vi "writegraph_OLD.vi"(4 "Numeric":i16, 5 "Array":string[][](array[string])) -> ()   [LabVIEW 2011]
uses:
  Dependencies/global.vi
panel:
  out "Humidity (Mote 1001)":dbl(graph)
  out "Temperature (Mote 1001)":dbl(graph)
  out "CO2 (Mote 1001)":dbl(graph)
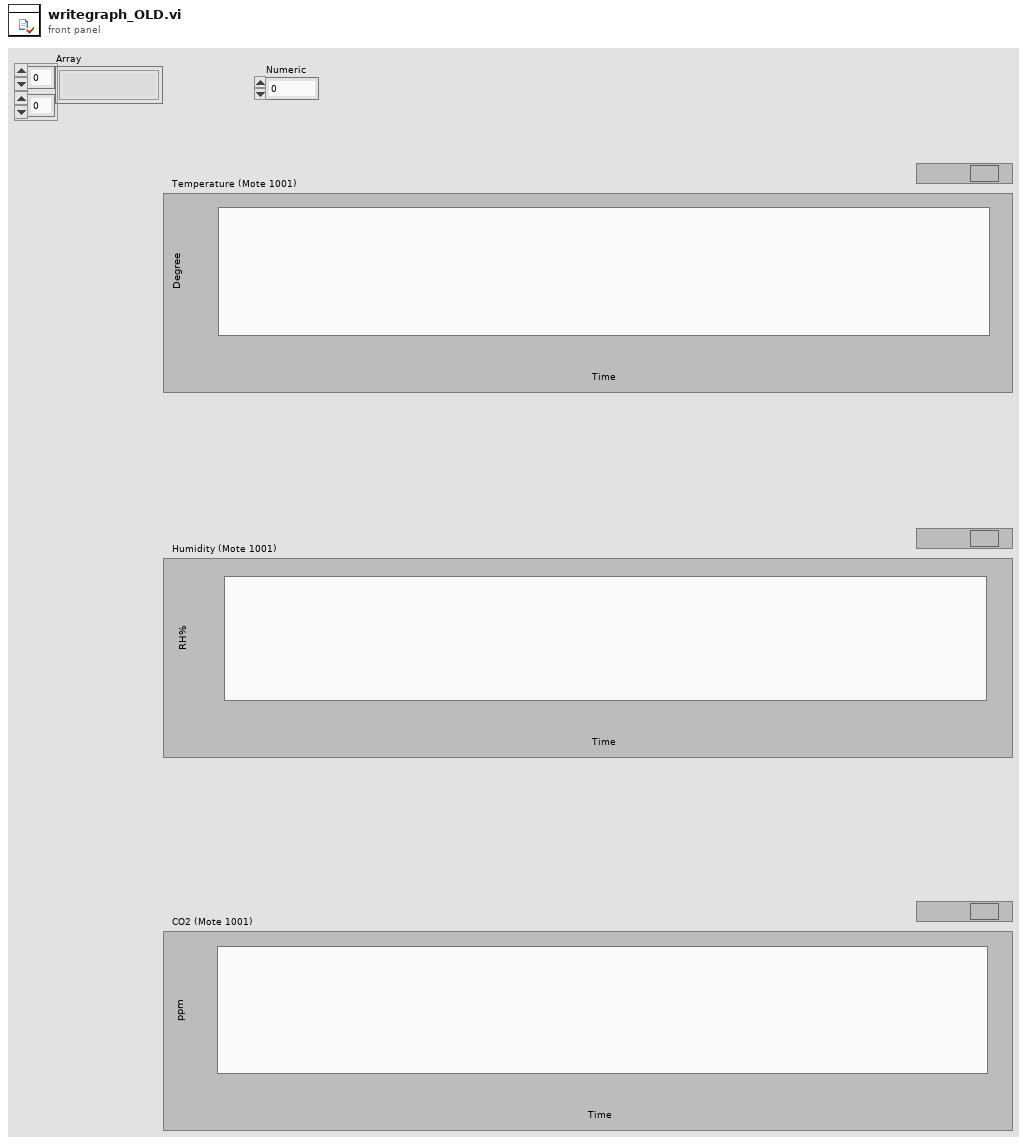
[diagram p1: front panel]
types:
  T1 = typedef "imagedata.ctl" = cluster{"image type":i32, "image depth":i32, "image":u8[], "mask":u8[], "colors":u32[], "Rectangle":cluster{"left":i16, "top":i16, "right":i16, "bottom":i16}}
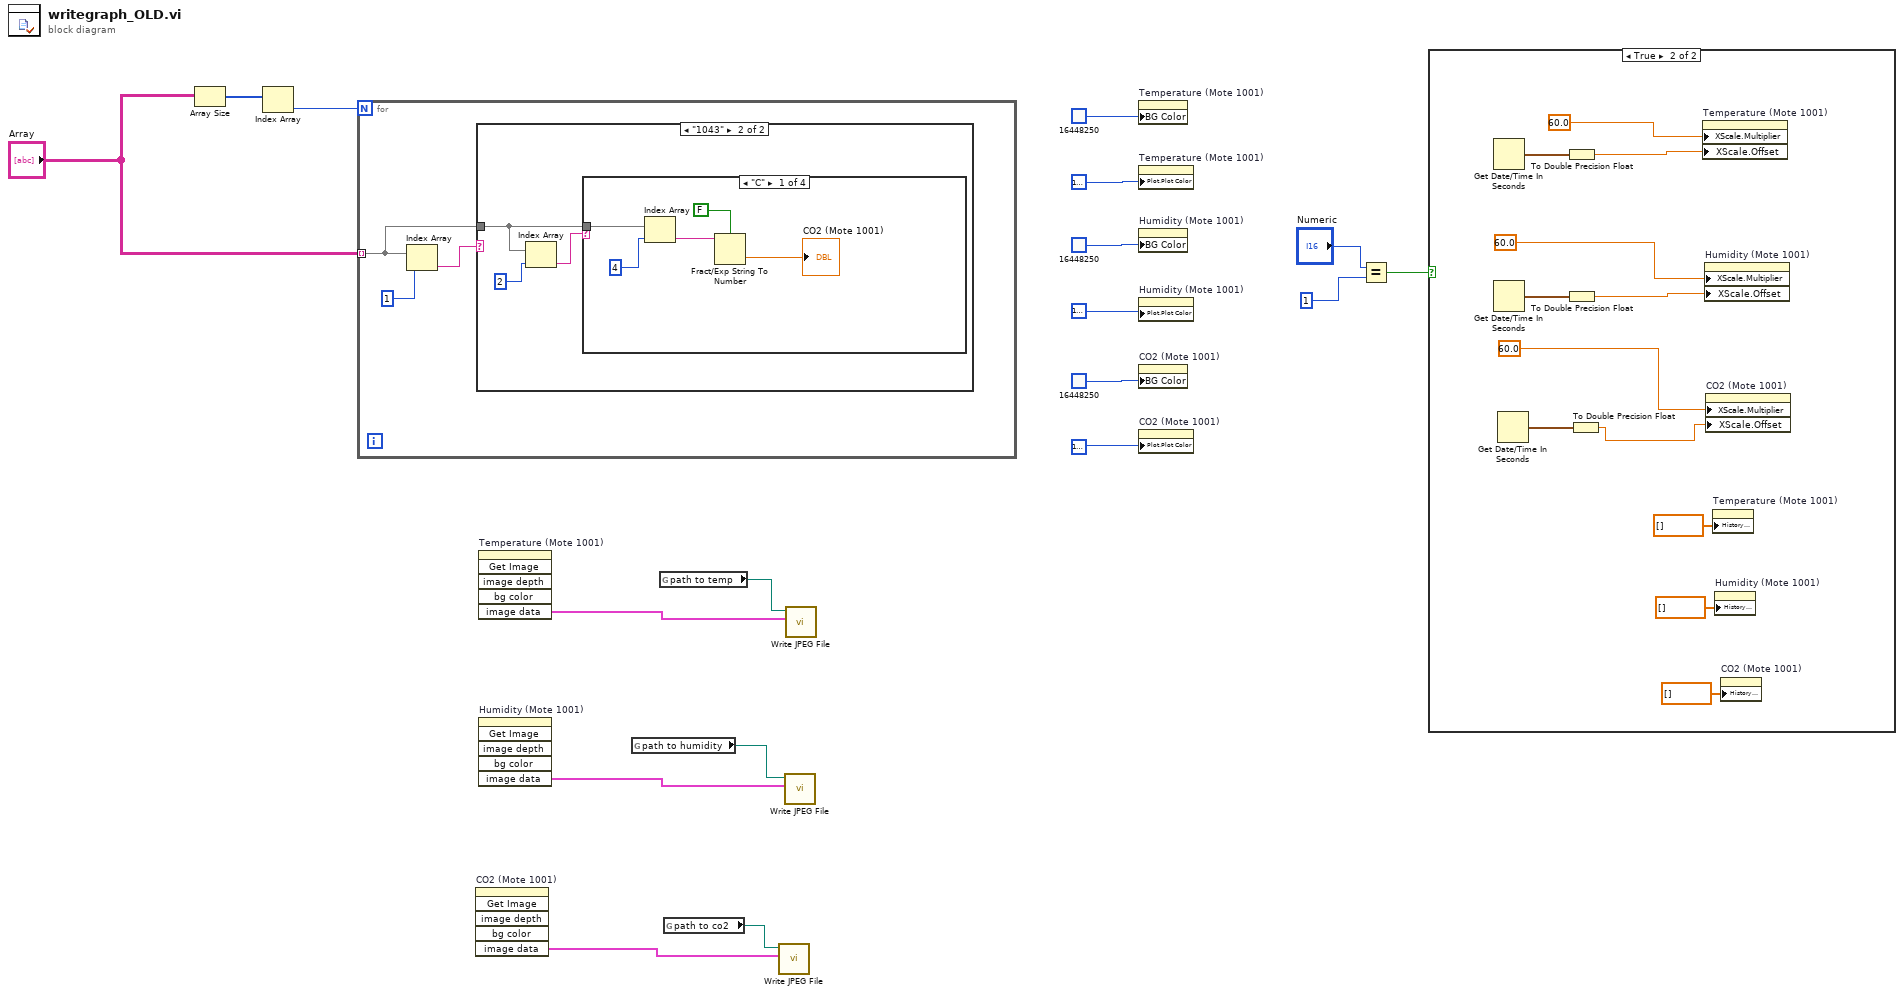
[diagram p0: block diagram]
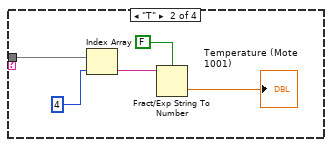
[diagram p4: hidden frame]
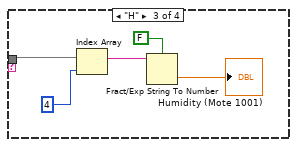
[diagram p5: hidden frame]
diagram:
  n1 = Array Size(array="Array") -> (size(s)=w18:i32[])
  n2 = Index Array(array=w18) -> (element=w17:i32)  [unwired: 1 in]
  n3 = for {
    N: w17 -> [_]
    tunnel: "Array" -> [w19] mode=indexing
    n4 = Index Array(array=w19, index=1) -> (element=w20:string)
    n5 = case shown="\"1043\"" w20 {
      tunnel: w19 -> [_ w24]
      frame "0", Default {
      }
      frame "1043" {
        n6 = Index Array(array=w24, index=2) -> (element=w22:string)
        n7 = case shown="\"C\"" w22 {
          tunnel: w24 -> [w27 w34 w37 _]
          frame "C" {
            n8 = Index Array(array=w27, index=4 ("index (row)")) -> (element=w28:string)
            n9 = Fract/Exp String To Number(use system decimal point (T)=FALSE, string=w28) -> (number=→"CO2 (Mote 1001)":dbl)  [unwired: 2 in, 1 out]
          }
          frame "T" {
            n10 = Index Array(array=w34, index=4 ("index (row)")) -> (element=w32:string)
            n11 = Fract/Exp String To Number(use system decimal point (T)=FALSE, string=w32) -> (number=→"Temperature (Mote 1001)":dbl)  [unwired: 2 in, 1 out]
          }
          frame "H" {
            n12 = Index Array(array=w37, index=4 ("index (row)")) -> (element=w38:string)
            n13 = Fract/Exp String To Number(use system decimal point (T)=FALSE, string=w38) -> (number=→"Humidity (Mote 1001)":dbl)  [unwired: 2 in, 1 out]
          }
          frame Default {
          }
        }
      }
    }
  }
  n14 = invoke on="CO2 (Mote 1001)" class="WFChart (strict)" method="Get Image"() -> ("image data"=w7:T1)  [unwired: 6 in, 5 out]
  n15 = invoke on="Temperature (Mote 1001)" class="WFChart (strict)" method="Get Image"() -> ("image data"=w9:T1)  [unwired: 6 in, 5 out]
  n16 = invoke on="Humidity (Mote 1001)" class="WFChart (strict)" method="Get Image"() -> ("image data"=w8:T1)  [unwired: 6 in, 5 out]
  n17 = global read "global.vi" "path to humidity"() -> (w2:path)
  n18 = global read "global.vi" "path to temp"() -> (w1:path)
  n19 = global read "global.vi" "path to co2"() -> (w3:path)
  n20 = call <vilib>:"Write JPEG File.vi"("image data"=w7, "path to JPEG file"=w3) -> ()  [unwired: 8 in, 2 out]
  n21 = call <vilib>:"Write JPEG File.vi"("image data"=w8, "path to JPEG file"=w2) -> ()  [unwired: 8 in, 2 out]
  n22 = call <vilib>:"Write JPEG File.vi"("image data"=w9, "path to JPEG file"=w1) -> ()  [unwired: 8 in, 2 out]
  n23 = property on="Temperature (Mote 1001)" class="WFChart (strict)"("BG Color"=u32 16448250) -> ()  [unwired: 2 in, 2 out]
  n24 = property on="Temperature (Mote 1001)" class="WFChart (strict)"("Plot.Plot Color"=u32 16777222) -> ()  [unwired: 2 in, 2 out]
  n25 = property on="Humidity (Mote 1001)" class="WFChart (strict)"("BG Color"=u32 16448250) -> ()  [unwired: 2 in, 2 out]
  n26 = property on="Humidity (Mote 1001)" class="WFChart (strict)"("Plot.Plot Color"=u32 16777222) -> ()  [unwired: 2 in, 2 out]
  n27 = property on="CO2 (Mote 1001)" class="WFChart (strict)"("BG Color"=u32 16448250) -> ()  [unwired: 2 in, 2 out]
  n28 = property on="CO2 (Mote 1001)" class="WFChart (strict)"("Plot.Plot Color"=u32 16777222) -> ()  [unwired: 2 in, 2 out]
  n29 = Equal?(x="Numeric", y=i16 1) -> (x = y?=w6:bool)
  n30 = case shown="True" w6 {
    frame False {
    }
    frame True {
      n31 = Get Date/Time In Seconds() -> (seconds since 1Jan1904=w51:timestamp)
      n32 = Get Date/Time In Seconds() -> (seconds since 1Jan1904=w50:timestamp)
      n33 = Get Date/Time In Seconds() -> (seconds since 1Jan1904=w48:timestamp)
      n34 = To Double Precision Float(number=w51) -> (double precision float=w45:dbl)
      n35 = To Double Precision Float(number=w50) -> (double precision float=w44:dbl)
      n36 = To Double Precision Float(number=w48) -> (double precision float=w43:dbl)
      n37 = property on="Temperature (Mote 1001)" class="WFChart (strict)"("XScale.Multiplier"=60.0 ("X Scale.Offset and Multiplier:Multiplier"), "XScale.Offset"=w45) -> ()  [unwired: 2 in, 2 out]
      n38 = property on="Humidity (Mote 1001)" class="WFChart (strict)"("XScale.Multiplier"=60.0 ("X Scale.Offset and Multiplier:Multiplier"), "XScale.Offset"=w44) -> ()  [unwired: 2 in, 2 out]
      n39 = property on="CO2 (Mote 1001)" class="WFChart (strict)"("XScale.Multiplier"=60.0 ("X Scale.Offset and Multiplier:Multiplier"), "XScale.Offset"=w43) -> ()  [unwired: 2 in, 2 out]
      n40 = property on="Temperature (Mote 1001)" class="WFChart (strict)"("History Data"=dbl[] []) -> ()  [unwired: 2 in, 2 out]
      n41 = property on="Humidity (Mote 1001)" class="WFChart (strict)"("History Data"=dbl[] []) -> ()  [unwired: 2 in, 2 out]
      n42 = property on="CO2 (Mote 1001)" class="WFChart (strict)"("History Data"=dbl[] []) -> ()  [unwired: 2 in, 2 out]
    }
  }
